vi "Window-Export time series images.vi"(10 "New folder path":path, 11 "Existing AVI path":path) -> ()   [LabVIEW 2020]
uses:
  <vilib>/Utility/miscctls.llb/LVPointTypeDef.ctl
  <vilib>/vision/NI_Vision_Development_Module.lvlib
panel:
  out "Ended":bool
  out "Manually closed":bool
  out "Exporting time-lapse images...":u8(slide) scale=0.0..100.0
  out "# of Frames in exported portion":i32 format="Number of frames: %.0f"
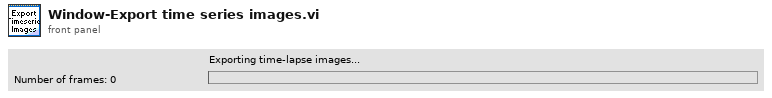
[diagram p1: front panel]
types:
  T1 = typedef "Image Type" = u32
  T2 = typedef "LVPointTypeDef.ctl" = cluster{"Horizontal":i16, "Vertical":i16}
  T3 = typedef "Fixed strings.ctl" = cluster{"ROI file name":string, "Normalised ROI file name":string, "Zplane Pockels values file name":string, "Functional data folder name":string, "Experiment Header file name":string, "Z-stack images folder name":string, "Groups setup rel. path":string, "Groups text file rel. path":string, "TDMS files folder name (F.img)":string, "TDMS files folder name (V.acq)":string, "TDMS files folder name (Pl.acq)":string, "Cycle rel times sequence file":string, "Dynamically called VIs folder name":string, "Time Series folder base name":string}
  T4 = typedef "AVI modes refs cluster.ctl" = cluster{"AVI1 ref":T5, "AVI2 refs":T6[], "AVI # frames":u32[]}
  T5 = typedef "AviRefnum.ctl" = refnum<k1>
  T6 = typedef "IMAQ AVI2 Refnum.ctl" = refnum<k20>
  T7 = typedef "IMAQ Image.ctl" = refnum<image>
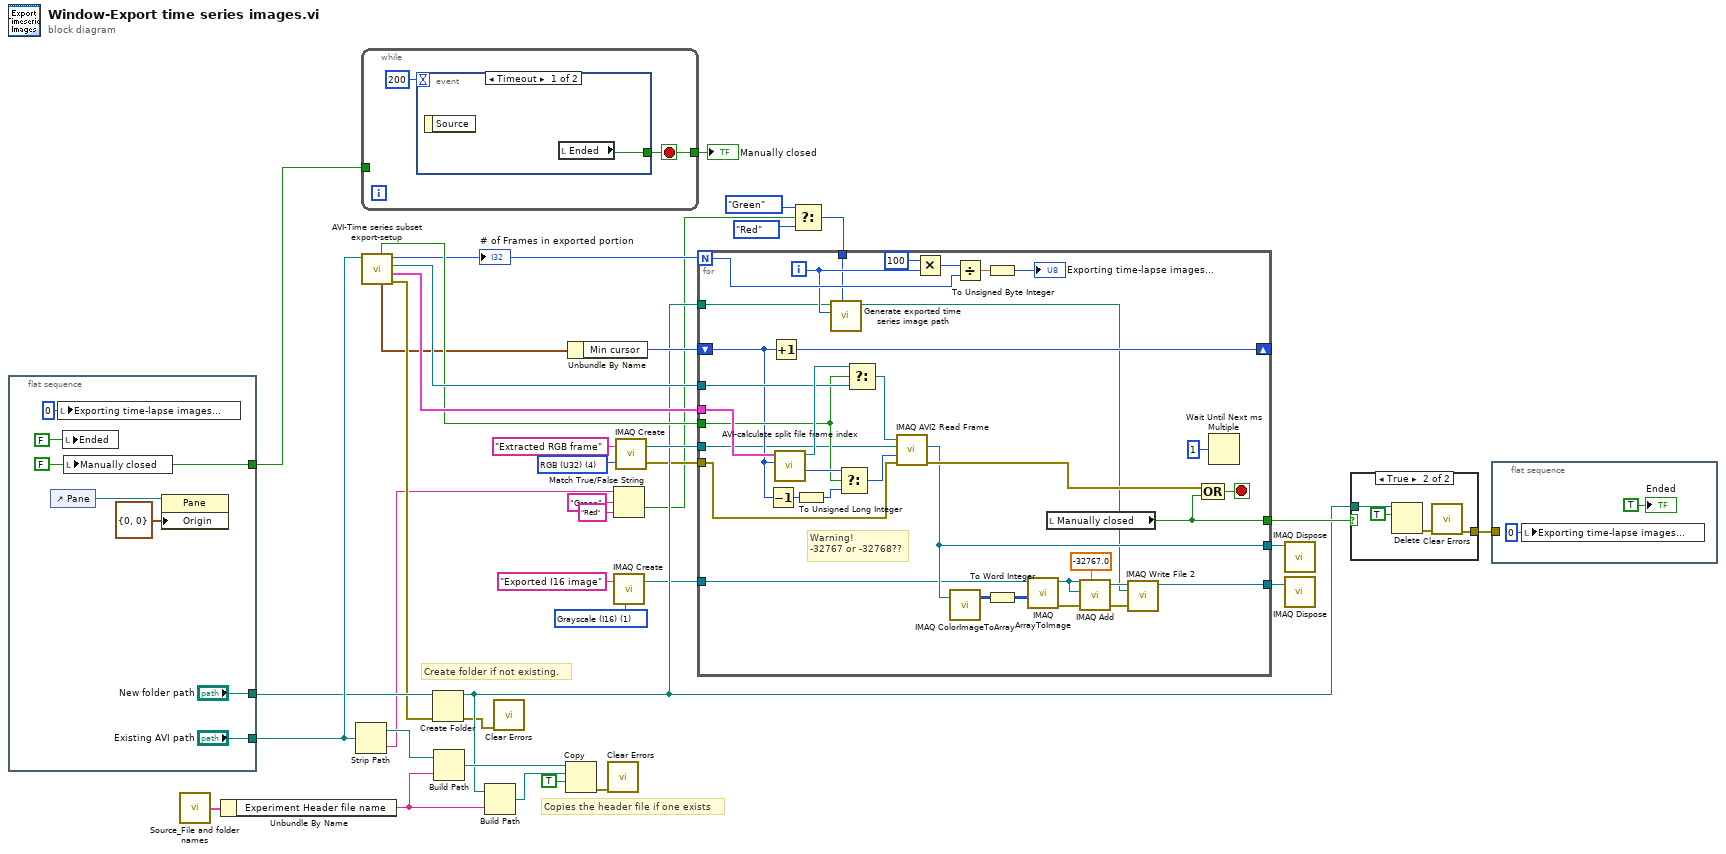
[diagram p0: block diagram]
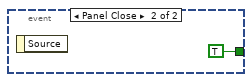
[diagram p3: hidden frame]
diagram:
  w14 = T1 1 items=["Grayscale (U8)", "Grayscale (I16)", "Grayscale (SGL)", "Complex (CSG)", "RGB (U32)", "HSL (U32)", "RGB (U64)", "Grayscale (U16)"] ("Image Type")
  w37 = T1 4 items=["Grayscale (U8)", "Grayscale (I16)", "Grayscale (SGL)", "Complex (CSG)", "RGB (U32)", "HSL (U32)", "RGB (U64)", "Grayscale (U16)"] ("Image Type")
  # "Create folder if not existing."
  # "Copies the header file if one exists"
  n1 = flat-sequence {
    tunnel: ["Existing AVI path"] -> w23
    tunnel: ["New folder path"] -> w22
    tunnel: [w43] -> w10
    frame #0 {
      w43 = FALSE
      n2 = control-ref of="Pane"() -> (w39:refnum<vi>)
      n3 = local write "Exporting time-lapse images..."(u8 0 ("Progress...")) -> ()
      n4 = local write "Ended"(FALSE) -> ()
      n5 = local write "Manually closed"(w43) -> ()
      n6 = property class="Pane"(reference=w39, "Origin"=T2 {"Horizontal"=0, "Vertical"=0}) -> ()  [unwired: 1 in, 2 out]
    }
  }
  n7 = call "Source_File and folder names.vi"() -> ("Fixed strings"=w6:T3)  [unwired: 1 in]
  n8 = Unbundle By Name(w6) -> ("Experiment Header file name"=w5:string)
  n9 = Strip Path(path=w23) -> (stripped path=w29:path, name=w16:string)
  n10 = while {
    tunnel: [w46] -> w38
    tunnel: w10 -> [_]
    stop <- w46 stop-if-true
    n11 = event shown="[0] Timeout" {
      selector: _ -> [_ _]
      dyn-events: _ -> [_ _]
      timeout: 200 -> [_ _]
      tunnel: [w48 TRUE] -> w46
      event Timeout {
        n12 = event-data() -> ()  [unwired: 1 in, 1 out]
        n13 = local read "Ended"() -> (w48:bool)
      }
      event Panel Close {
        n14 = event-data() -> ()  [unwired: 1 in, 1 out]
      }
    }
  }
  "Manually closed" <- w38
  n15 = call "AVI-Time series subset export-setup.vi"("AVI path & name"=w23) -> ("error out"=w21:errorcluster, "AVI modes refs"=w35:T4, "AVI Refnum (duplicate)"=w33:T6, "# of Frames in exported portion"=w20:i32, "Extraction cursors"=w19:cluster{"Min cursor":i32, "Max cursor":i32}, "Export all split AVI files as one"=w24:bool)  [unwired: 5 in]
  "# of Frames in exported portion" <- w20
  n16 = Create Folder(path (use dialog)=w22, error in=w21) -> (created path=w15:path, error out=w7:errorcluster)  [unwired: 1 in, 1 out]
  n17 = Build Path(base path=w29, name or relative path=w5) -> (appended path=w28:path)
  n18 = Build Path(base path=w15, name or relative path=w5) -> (appended path=w27:path)
  n19 = call <vilib>:"Clear Errors.vi"("error in (no error)"=w7) -> ()  [unwired: 5 in, 2 out]
  n20 = Copy(9:TRUE ("overwrite (F)"), 10:w27, 11:w28) -> (0:w8:errorcluster)  [unwired: 2 in, 2 out]
  n21 = Unbundle By Name(w19) -> ("Min cursor"=w32:i32)
  n22 = call <vilib>:"Clear Errors.vi"("error in (no error)"=w8) -> ()  [unwired: 5 in, 2 out]
  n23 = Match True/False String(2:"Red" ("false string"), 3:"Green" ("pattern"), 4:w16) -> (0:w4:bool)  [unwired: 1 out]
  n24 = call "IMAQ Create"("Image Name"="Exported I16 image", "Image Type"=w14) -> ("New Image"=w12:T7)  [unwired: 2 in, 2 out]
  n25 = call "IMAQ Create"("Image Name"="Extracted RGB frame", "Image Type"=w37) -> ("New Image"=w34:T7, "error out"=w9:errorcluster)  [unwired: 2 in, 1 out]
  n26 = Select(t=enum16{"Green", "Red"}."Green" ("Channel"), s=w4, f=enum16{"Green", "Red"}."Red" ("Channel")) -> (s? t:f=w1:enum16{"Green", "Red"})
  n27 = for {
    N: w20 -> [w73]
    tunnel: w33 -> [w83]
    tunnel: w34 -> [w70]
    tunnel: w35 -> [w85]
    tunnel: w24 -> [w81]
    shift-right: [w71] -> _
    shift-left: w32 -> [w72]
    tunnel: [w63] -> w31
    tunnel: [w65] -> w30
    tunnel: w1 -> [w56]
    tunnel: w15 -> [w55]
    tunnel: w12 -> [w53]
    tunnel: [w52] -> w11
    tunnel: w9 -> [w50]
    i -> [w57]
    stop <- w80 stop-if-true
    # "Warning!\n-32767 or -32768??"
    n28 = Decrement(x=w72) -> (x-1=w75:i32)
    n29 = Increment(x=w72) -> (x+1=w71:i32)
    n30 = call "AVI-calculate split file frame index.vi"("Frame number (unity-based) in"=w72, "AVI modes refs"=w85) -> ("Index of frame in split file"=w82:u32, "AVI2 split file ref"=w84:T6)  [unwired: 6 in, 2 out]
    n31 = To Unsigned Long Integer(number=w75) -> (unsigned 32bit integer=w74:u32)
    n32 = call "Generate exported time series image path.vi"("Channel"=w56, "FOR loop iteration"=w57, "Folder path"=w55) -> ("File path"=w54:path)  [unwired: 8 in]
    n33 = Select(t=w82, s=w81, f=w74) -> (s? t:f=w68:u32)
    n34 = Select(t=w84, s=w81, f=w83) -> (s? t:f=w69:T6)
    n35 = call "IMAQ AVI2 Read Frame"("error in (no error)"=w50, "Frame Number"=w68, "Image"=w70, "AVI Refnum"=w69) -> ("error out"=w67:errorcluster, "Image Out"=w63:T7)  [unwired: 5 in, 1 out]
    n36 = Multiply(x=100, y=w57) -> (x*y=w78:i32)
    n37 = call "IMAQ ColorImageToArray"("Image"=w63) -> ("Image Pixels (U32)"=w64:u32[][])  [unwired: 2 in, 3 out]
    n38 = Divide(x=w78, y=w73) -> (x/y=w77:dbl)
    n39 = To Unsigned Byte Integer(number=w77) -> (unsigned 8bit integer=→"Exporting time-lapse images...":u8)
    n40 = To Word Integer(number=w64) -> (16bit integer=w58:i16[][])
    n41 = call "IMAQ ArrayToImage"("Image Pixels (I16)"=w58, "Image"=w53) -> ("error out"=w60:errorcluster, "Image Out"=w51:T7)  [unwired: 8 in]
    n42 = local read "Manually closed"() -> (w65:bool)
    n43 = call "IMAQ Add"("Image Src A"=w51, "Constant"=-32767.0, "Image Dst"=w51, "error in (no error)"=w60) -> ("Image Dst Out"=w62:T7, "error out"=w61:errorcluster)  [unwired: 3 in]
    n44 = call-poly "IMAQ Write File 2"("error in (no error)"=w61, "File Path"=w54, "Image"=w62) -> ("Image Out (duplicate)"=w52:T7)  [unwired: 7 in, 1 out]
    n45 = Compound Arithmetic op=OR(w67, w65) -> (w80:bool)
    n46 = Wait Until Next ms Multiple(millisecond multiple=u32 1) -> ()  [unwired: 1 out]
  }
  n47 = call "IMAQ Dispose"("Image"=w31) -> ()  [unwired: 5 in, 1 out]
  n48 = call "IMAQ Dispose"("Image"=w11) -> ()  [unwired: 5 in, 1 out]
  n49 = case shown="True" w30 {
    tunnel: w15 -> [_ w89]
    tunnel: [_ w86] -> w25
    frame False {
    }
    frame True {
      n50 = Delete(path (use dialog)=w89, entire hierarchy (F)=TRUE) -> (error out=w88:errorcluster)  [unwired: 3 in, 2 out]
      n51 = call <vilib>:"Clear Errors.vi"("error in (no error)"=w88) -> ("error out"=w86:errorcluster)  [unwired: 5 in, 1 out]
    }
  }
  n52 = flat-sequence {
    tunnel: w25 -> [_]
    frame #0 {
      n53 = local write "Exporting time-lapse images..."(u8 0 ("Progress...")) -> ()
      "Ended" <- TRUE ("Ended")
    }
  }
